vi "[RT]GetStateRQST.vi"(11 "Queue in":refnum<queue>) -> (1 "target-temp":dbl, 3 "State Rqst":T1)   [LabVIEW 2018]
uses:
  TypeDef/ControllerState.ctl
  TypeDef/CMD Cluster.ctl
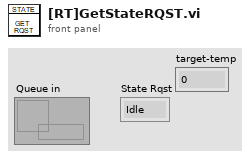
[diagram p1: front panel]
types:
  T1 = typedef "ControllerState.ctl" = enum16{"Idle", "Heizen", "Pumpen", "Emergency-Stop"}
  T2 = typedef "CMD Cluster.ctl" = cluster{"State Rqst":T1, "timestamp":u32, "temp":dbl}
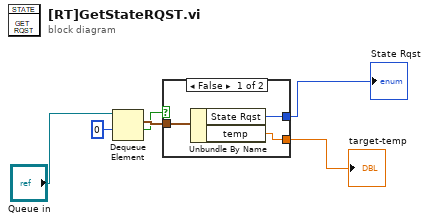
[diagram p0: block diagram]
diagram:
  n1 = Dequeue Element(queue="Queue in", timeout in ms (-1)=0) -> (element=w5:T2, timed out?=w4:bool)  [unwired: 1 in, 2 out]
  n2 = case shown="False" w4 {
    tunnel: w5 -> [w9 _]
    tunnel: [w8 _] -> w6
    tunnel: [w7 _] -> w1
    frame False {
      n3 = Unbundle By Name(w9) -> ("State Rqst"=w8:T1, "temp"=w7:dbl)
    }
    frame True {
    }
  }
  "State Rqst" <- w6
  "target-temp" <- w1
